vi "SetStationFullName.vi"(8 "error in":errorcluster, 10 "StationFullName":string, 11 "OperationRun in":refnum<class "OperationRun.lvclass">) -> (0 "error out":errorcluster, 3 "OperationRun out":refnum<class "OperationRun.lvclass">)   [LabVIEW 2021, in "ProligentXMLGenerator.lvlib" / "OperationRun.lvclass"]
doc: "Defines the station where the operation run was executed.\n\nThis attribute cannot be updated."
uses:
  OperationRun.lvclass
  OperationRun.lvclass/OperationRun.ctl
  Base/Attribute/Attribute.lvclass
  Base/FullName/FullName.lvclass
  C:/Projects/proligent-xml-generator-labview/src/ProligentXMLGenerator/Base/NonEmptyString/NonEmptyString.lvclass
  C:/Projects/proligent-xml-generator-labview/src/ProligentXMLGenerator/Base/String/String.lvclass
  C:/Projects/proligent-xml-generator-labview/src/ProligentXMLGenerator/Base/Attribute/Attribute.lvclass
  C:/Projects/proligent-xml-generator-labview/src/ProligentXMLGenerator/Base/FullName/FullName.lvclass
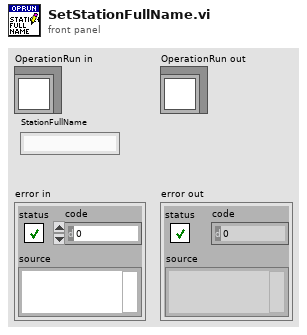
[diagram p1: front panel]
types:
  T1 = typedef "ProligentXMLGenerator.lvlib/OperationRun.lvclass/Data.ctl" = cluster{"Name":string, "Characteristics":refnum<class "Characteristic.lvclass">[], "Documents":refnum<class "Document.lvclass">[], "SequenceRuns":refnum<class "SequenceRun.lvclass">[], "FailureReferences":refnum<class "FailureReference.lvclass">[], "SequenceRunReferences":refnum<class "SequenceRunReference.lvclass">[], "CustomData":refnum<class "CustomData.lvclass">, "OperationRunId":refnum<class "Guid.lvclass">, "ProcessFullName":refnum<class "ProcessFullName.lvclass">, "ProcessVersion":refnum<class "NonEmptyString_64.lvclass">, "OperationName":refnum<class "NonEmptyString_65.lvclass">, "StationFullName":refnum<class "FullName.lvclass">, "User":refnum<class "NonEmptyString_255.lvclass">, "CallingOperationRunId":refnum<class "Guid.lvclass">, "OperationStatus":refnum<class "ExecutionStatus.lvclass">, "OperationRunStartTime":refnum<class "DateTime.lvclass">, "OperationRunEndTime":refnum<class "DateTime.lvclass">, "TimeZoneInfoId":string}
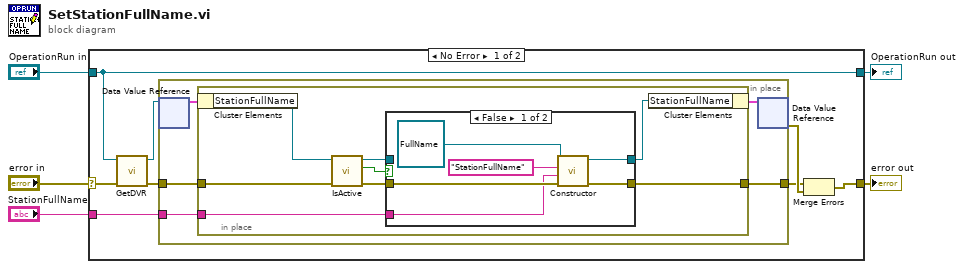
[diagram p0: block diagram]
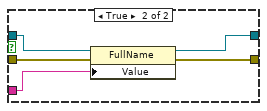
[diagram p2: hidden frame]
diagram:
  n1 = case shown="No Error" "error in" {
    selector: "error in" -> [w11 w38]
    tunnel: "OperationRun in" -> [w6 w39]
    tunnel: [w8 w38] -> w3
    tunnel: "StationFullName" -> [w7 _]
    tunnel: [w6 w39] -> w1
    frame No Error {
      n2 = call "GetDVR.vi"("error in"=w11, "OperationRun"=w6) -> ("error out"=w10:errorcluster, "DVRReference"=w12:refnum<data-value>)  [unwired: 8 in]
      n3 = in-place "In Place Element Structure" {
        in-place-border: w10 -> [w18]
        in-place-border: [w17] -> w9
        in-place-border: w7 -> [w16]
        n4 = in-place-dvr #1(w12) -> (w15:T1)  [unwired: 1 out]
        n5 = in-place "In Place Element Structure" {
          in-place-border: w18 -> [w22]
          in-place-border: [w26] -> w17
          in-place-border: w16 -> [w25]
          n6 = in-place-cluster #2(w15) -> ("StationFullName"=w21:refnum<class "FullName.lvclass">)
          n7 = call "IsActive.vi"("error in"=w22, "Attribute in"=w21) -> ("error out"=w23:errorcluster, "IsActive"=w19:bool, "Attribute in"=w20:refnum<class "FullName.lvclass">)  [unwired: 7 in]
          n8 = case shown="False" w19 {
            tunnel: w23 -> [w29 w37]
            tunnel: [w32 w36] -> w26
            tunnel: w25 -> [w28 w35]
            tunnel: [w31 w34] -> w24
            tunnel: w20 -> [_ w33]
            frame False {
              n9 = call-dynamic "Constructor.vi"("error in"=w29, "Value"=w28, "Name"="StationFullName", "String in"=refnum<class "FullName.lvclass"> refnum ("ProcessVersion")) -> ("error out"=w32:errorcluster, "String out"=w31:refnum<class "FullName.lvclass">)  [unwired: 6 in]
            }
            frame True {
              n10 = property on="Property Node" class="FullName"(reference=w33, error in=w37, "Value"=w35) -> (reference out=w34:refnum<class "FullName.lvclass">, error out=w36:errorcluster)
            }
          }
          n11 = in-place-cluster #2("StationFullName"=w24) -> (w14:T1)
        }
        n12 = in-place-dvr #1(w14) -> (w13:errorcluster)  [unwired: 1 out]
      }
      n13 = Merge Errors(w9, w13) -> (w8:errorcluster)
    }
    frame Error {
    }
  }
  "error out" <- w3
  "OperationRun out" <- w1
